vi "Calculate Sinusoidal Fit.vi"(4 "Offset":dbl format="%#_13g", 6 "Ignore Offset":bool, 9 "Sample Rate":i32, 10 "Stimulus\nFrequency":dbl=nan, 11 "Data in":dbl[](array[numeric])) -> (2 "Best Fit":dbl[](array[numeric]), 3 "Coefficients":T1 {"Freq" format="%#.2f"; "Offset" format="%.3f"; "Gain" format="%.2f"; "Phase" format="%.1f"})   [LabVIEW 2014, in "Sinusoidal Fit.lvclass"]
uses:
  Sinusoidal Fit.lvclass
  gain and phase/Typedef - Sinusoidal Fit Coefficients.ctl
  <vilib>/Analysis/NI_AALPro.lvlib
  Abstract Fit/Abstract Fit.lvclass
panel:
  out "Waveform Graph":dbl[][](graph)
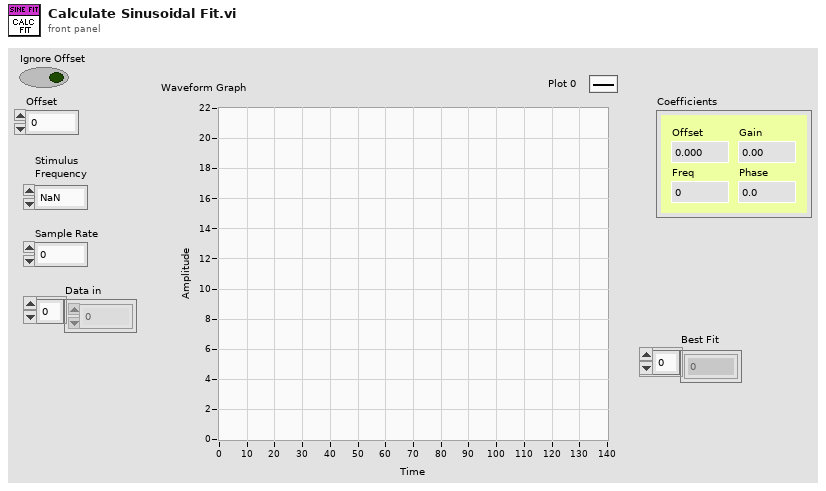
[diagram p1: front panel]
types:
  T1 = typedef "Typedef - Sinusoidal Fit Coefficients.ctl" = cluster{"Offset":dbl, "Gain":dbl, "Phase":dbl, "Freq":dbl}
  T2 = cluster{dbl, dbl, dbl, "Fundamental frequency":dbl}
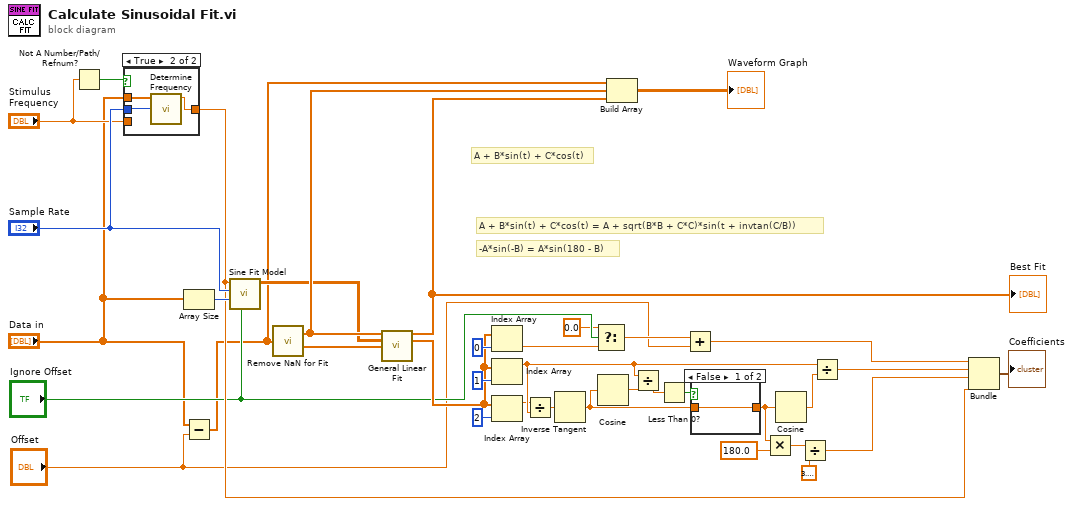
[diagram p0: block diagram]
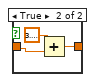
[diagram p3: hidden frame]
diagram:
  # "A + B*sin(t) + C*cos(t) = A + sqrt(B*B + C*C)*sin(t + invtan(C/B))"
  # "A + B*sin(t) + C*cos(t)"
  # "-A*sin(-B) = A*sin(180 - B)"
  n1 = Not A Number/Path/Refnum?(number/path/refnum="Stimulus\nFrequency") -> (NaN/Path/Refnum?=w13:bool)
  n2 = case shown="True" w13 {
    tunnel: [w38 w40] -> w14
    tunnel: "Stimulus\nFrequency" -> [w38 _]
    tunnel: "Data in" -> [_ w41]
    tunnel: "Sample Rate" -> [_ w39]
    frame False {
    }
    frame True {
      n3 = call "Determine Frequency.vi"("Sample Rate"=w39, "Signal (in)"=w41) -> ("Fundamental frequency"=w40:dbl)  [unwired: 5 in]
    }
  }
  n4 = Array Size(array="Data in") -> (size(s)=w22:i32)
  n5 = Subtract(x="Data in", y="Offset") -> (x-y=w4:dbl[])
  n6 = call "Sine Fit Model.vi"("Ignore Offset"="Ignore Offset", "Length"=w22, "Sample Rate"="Sample Rate", "Frequency"=w14) -> ("Array"=w9:ext[][])  [unwired: 7 in]
  n7 = call "Remove NaN for Fit.vi"("Data in"=w4) -> ("Weight out"=w10:dbl[], "Data out"=w11:dbl[])  [unwired: 2 in]
  n8 = call <vilib>:"General Linear Fit.vi"("Y"=w11, "H"=w9, "Weight"=w10) -> ("Best Fit"=w17:dbl[], "Coefficients"=w21:dbl[])  [unwired: 7 in, 4 out]
  "Best Fit" <- w17
  n9 = Index Array(array=w21, index=0 ("Index")) -> (element=w7:dbl)
  n10 = Index Array(array=w21, index=1 ("Index")) -> (element=w34:dbl)
  n11 = Index Array(array=w21, index=2 ("Index")) -> (element=w26:dbl)
  n12 = Divide(x=w26, y=w34) -> (x/y=w31:dbl)
  n13 = Inverse Tangent(1:w31) -> (0:w33:dbl)
  n14 = Select(t=0.0, s="Ignore Offset", f=w7) -> (s? t:f=w3:dbl)
  n15 = Cosine(x=w33) -> (cos(x)=w35:dbl)
  n16 = Build Array(w4, w11, w17) -> (→"Waveform Graph":dbl[][])
  n17 = Divide(x=w34, y=w35) -> (x/y=w37:dbl)
  n18 = Less Than 0?(x=w37) -> (x < 0?=w36:bool)
  n19 = Add(x=w3, y="Offset") -> (x+y=w2:dbl)
  n20 = case shown="False" w36 {
    tunnel: w33 -> [w42 w44]
    tunnel: [w42 w43] -> w32
    frame False {
    }
    frame True {
      n21 = Add(x=3.141592653589793, y=w44) -> (x+y=w43:dbl)
    }
  }
  n22 = Multiply(x=w32, y=180.0) -> (x*y=w30:dbl)
  n23 = Cosine(x=w32) -> (cos(x)=w27:dbl)
  n24 = Divide(x=w30, y=3.141592653589793) -> (x/y=w19:dbl)
  n25 = Divide(x=w34, y=w27) -> (x/y=w20:dbl)
  n26 = Bundle(w2, w20, w19, "Fundamental frequency"=w14) -> (→"Coefficients":T2)  [unwired: 1 in]
